vi "Plan All Autonomous Drive Trajectories.vi"   [LabVIEW 2015]
uses:
  Autonomous Trajectories.vi
types:
  T1 = cluster{"Length":dbl, "Time":dbl, "Center":cluster{"Velocity":dbl, "Accel":dbl}, "Left":cluster{"Velocity":dbl, "Accel":dbl}, "Right":cluster{"Velocity":dbl, "Accel":dbl}, "Pose":cluster{"X":dbl, "Y":dbl, "Theta[rad]":dbl}}[]
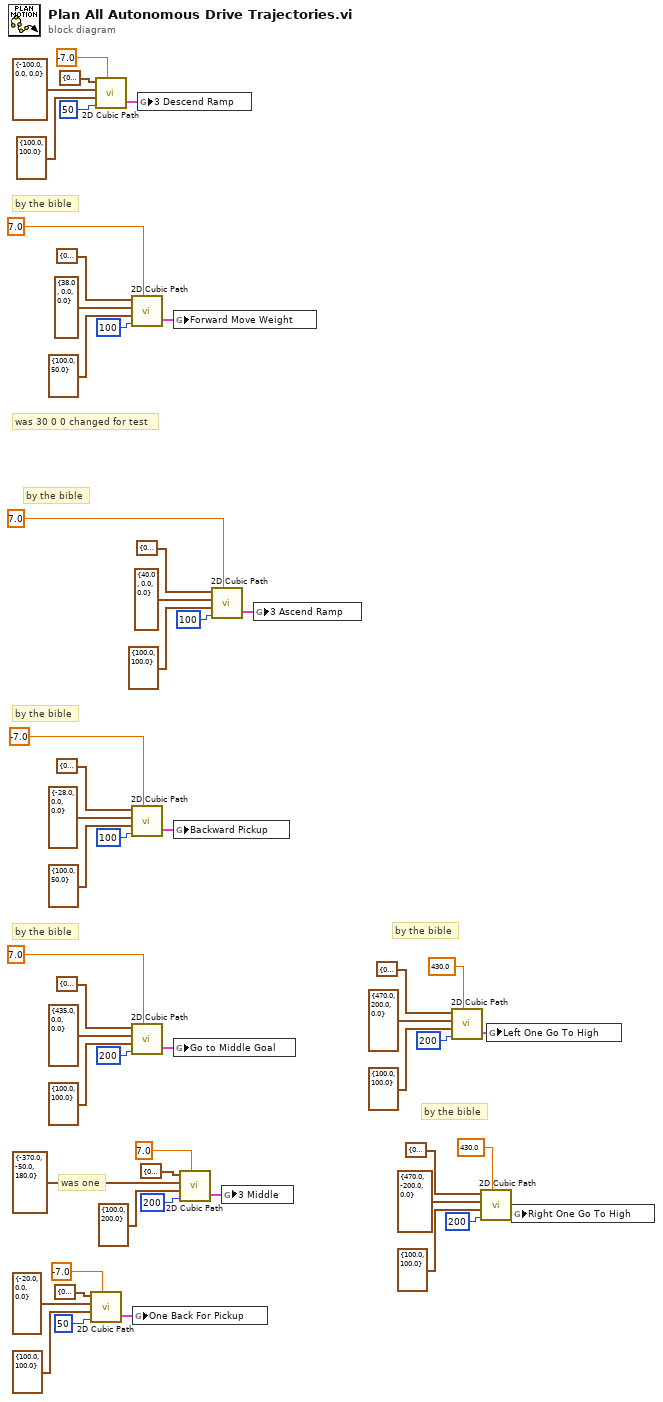
[diagram p0: block diagram]
diagram:
  # "by the bible"
  # "by the bible"
  # "was one"
  # "by the bible"
  # "by the bible"
  # "by the bible"
  # "was 30 0 0 changed for test"
  # "by the bible"
  n1 = call "2D Cubic Path.vi"("Pose i"=cluster{"X":dbl, "Y":dbl, "Theta[deg]":dbl} {"X"=0.0, "Y"=0.0, "Theta[deg]"=0.0}, "Pose f"=cluster{"X":dbl, "Y":dbl, "Theta[deg]":dbl} {"X"=-20.0, "Y"=0.0, "Theta[deg]"=0.0}, "Constraints"=cluster{"Vmax":dbl, "Amax":dbl} {"Vmax"=100.0, "Amax"=100.0}, "Number Of Points"=50, "K"=-7.0) -> ("Motion Profile"=w37:T1)  [unwired: 1 out]
  n2 = call "2D Cubic Path.vi"("Pose i"=cluster{"X":dbl, "Y":dbl, "Theta[deg]":dbl} {"X"=0.0, "Y"=0.0, "Theta[deg]"=0.0}, "Pose f"=cluster{"X":dbl, "Y":dbl, "Theta[deg]":dbl} {"X"=-100.0, "Y"=0.0, "Theta[deg]"=0.0}, "Constraints"=cluster{"Vmax":dbl, "Amax":dbl} {"Vmax"=100.0, "Amax"=100.0}, "Number Of Points"=50, "K"=-7.0) -> ("Motion Profile"=w43:T1)  [unwired: 1 out]
  n3 = call "2D Cubic Path.vi"("Pose i"=cluster{"X":dbl, "Y":dbl, "Theta[deg]":dbl} {"X"=0.0, "Y"=0.0, "Theta[deg]"=0.0}, "Pose f"=cluster{"X":dbl, "Y":dbl, "Theta[deg]":dbl} {"X"=38.0, "Y"=0.0, "Theta[deg]"=0.0}, "Constraints"=cluster{"Vmax":dbl, "Amax":dbl} {"Vmax"=100.0, "Amax"=50.0}, "Number Of Points"=100, "K"=7.0) -> ("Motion Profile"=w31:T1)  [unwired: 1 out]
  n4 = call "2D Cubic Path.vi"("Pose i"=cluster{"X":dbl, "Y":dbl, "Theta[deg]":dbl} {"X"=0.0, "Y"=0.0, "Theta[deg]"=0.0}, "Pose f"=cluster{"X":dbl, "Y":dbl, "Theta[deg]":dbl} {"X"=-28.0, "Y"=0.0, "Theta[deg]"=0.0}, "Constraints"=cluster{"Vmax":dbl, "Amax":dbl} {"Vmax"=100.0, "Amax"=50.0}, "Number Of Points"=100, "K"=-7.0) -> ("Motion Profile"=w25:T1)  [unwired: 1 out]
  n5 = call "2D Cubic Path.vi"("Pose i"=cluster{"X":dbl, "Y":dbl, "Theta[deg]":dbl} {"X"=0.0, "Y"=0.0, "Theta[deg]"=0.0}, "Pose f"=cluster{"X":dbl, "Y":dbl, "Theta[deg]":dbl} {"X"=435.0, "Y"=0.0, "Theta[deg]"=0.0}, "Constraints"=cluster{"Vmax":dbl, "Amax":dbl} {"Vmax"=100.0, "Amax"=100.0}, "Number Of Points"=200, "K"=7.0) -> ("Motion Profile"=w19:T1)  [unwired: 1 out]
  n6 = global write "Autonomous Trajectories.vi" "One Back For Pickup"(w37) -> ()
  n7 = global write "Autonomous Trajectories.vi" "3 Descend Ramp"(w43) -> ()
  n8 = global write "Autonomous Trajectories.vi" "Forward Move Weight"(w31) -> ()
  n9 = global write "Autonomous Trajectories.vi" "Backward Pickup"(w25) -> ()
  n10 = global write "Autonomous Trajectories.vi" "Go to Middle Goal"(w19) -> ()
  n11 = call "2D Cubic Path.vi"("Pose i"=cluster{"X":dbl, "Y":dbl, "Theta[deg]":dbl} {"X"=0.0, "Y"=0.0, "Theta[deg]"=0.0}, "Pose f"=cluster{"X":dbl, "Y":dbl, "Theta[deg]":dbl} {"X"=-370.0, "Y"=-50.0, "Theta[deg]"=180.0}, "Constraints"=cluster{"Vmax":dbl, "Amax":dbl} {"Vmax"=100.0, "Amax"=200.0}, "Number Of Points"=200, "K"=7.0) -> ("Motion Profile"=w14:T1)  [unwired: 1 out]
  n12 = call "2D Cubic Path.vi"("Pose i"=cluster{"X":dbl, "Y":dbl, "Theta[deg]":dbl} {"X"=0.0, "Y"=0.0, "Theta[deg]"=0.0}, "Pose f"=cluster{"X":dbl, "Y":dbl, "Theta[deg]":dbl} {"X"=40.0, "Y"=0.0, "Theta[deg]"=0.0}, "Constraints"=cluster{"Vmax":dbl, "Amax":dbl} {"Vmax"=100.0, "Amax"=100.0}, "Number Of Points"=100, "K"=7.0) -> ("Motion Profile"=w49:T1)  [unwired: 1 out]
  n13 = global write "Autonomous Trajectories.vi" "3 Middle"(w14) -> ()
  n14 = global write "Autonomous Trajectories.vi" "3 Ascend Ramp"(w49) -> ()
  n15 = call "2D Cubic Path.vi"("Pose i"=cluster{"X":dbl, "Y":dbl, "Theta[deg]":dbl} {"X"=0.0, "Y"=0.0, "Theta[deg]"=0.0}, "Pose f"=cluster{"X":dbl, "Y":dbl, "Theta[deg]":dbl} {"X"=470.0, "Y"=200.0, "Theta[deg]"=0.0}, "Constraints"=cluster{"Vmax":dbl, "Amax":dbl} {"Vmax"=100.0, "Amax"=100.0}, "Number Of Points"=200, "K"=430.0) -> ("Motion Profile"=w7:T1)  [unwired: 1 out]
  n16 = call "2D Cubic Path.vi"("Pose i"=cluster{"X":dbl, "Y":dbl, "Theta[deg]":dbl} {"X"=0.0, "Y"=0.0, "Theta[deg]"=0.0}, "Pose f"=cluster{"X":dbl, "Y":dbl, "Theta[deg]":dbl} {"X"=470.0, "Y"=-200.0, "Theta[deg]"=0.0}, "Constraints"=cluster{"Vmax":dbl, "Amax":dbl} {"Vmax"=100.0, "Amax"=100.0}, "Number Of Points"=200, "K"=430.0) -> ("Motion Profile"=w1:T1)  [unwired: 1 out]
  n17 = global write "Autonomous Trajectories.vi" "Left One Go To High"(w7) -> ()
  n18 = global write "Autonomous Trajectories.vi" "Right One Go To High"(w1) -> ()
